vi "System config window - standalone.vi"   [LabVIEW 2020]
uses:
  Typedefs/Save-Load enum.ctl
  Typedefs/HW config states enum.ctl
types:
  T1 = typedef "HW config states enum.ctl" = enum16{"Load from file", "Save to file", "Save backup", "Write all", "Read all", "Write XY stage settings", "Write DAQ FPGA settings", "Write Control FPGA settings", "Write Phys Channels", "Write System Config", "Write HW Config", "Save System Config", "Save HW Config", "Clear", "Compare from file"}
  T2 = typedef "Save-Load enum.ctl" = enum16{"Save to file", "Load from file", "Compare from file", "Save Backup"}
  T3 = enum16{"Initialise", "Load from file", "Save to file", "Read", "Write"}
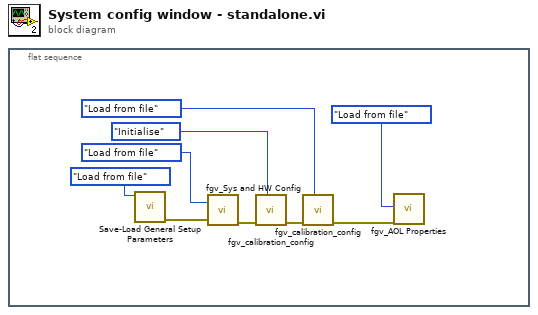
[diagram p0: block diagram]
diagram:
  n1 = flat-sequence {
    frame #0 {
      n2 = call "Save-Load General Setup Parameters.vi"("Function"=Save-Load_enum."Load from file") -> ("error out"=w3:errorcluster)  [unwired: 10 in]
      n3 = call "fgv_Sys and HW Config.vi"("Function"=HW_config_states_enum."Load from file", "error in (no error)"=w3) -> ("error out"=w5:errorcluster)  [unwired: 7 in, 2 out]
      n4 = call "fgv_calibration_config.vi"("Cal config ops"=T3."Initialise", "error in (no error)"=w5) -> ("error out"=w7:errorcluster)  [unwired: 7 in, 2 out]
      n5 = call "fgv_calibration_config.vi"("Cal config ops"=T3."Load from file", "error in (no error)"=w7) -> ("error out"=w1:errorcluster)  [unwired: 7 in, 2 out]
      n6 = call "fgv_AOL Properties.vi"("error in (no error)"=w1, "Function"=HW_config_states_enum."Load from file") -> ()  [unwired: 8 in, 2 out]
    }
  }
